vi "RT Connection.vi"(9 "Next State in":T1, 10 "reader endpoint":refnum<k21>, 11 "writer endpoint":refnum<k21>) -> (1 "Next State out":T1)   [LabVIEW 2021]
uses:
  Controls/RT Network States.ctl
  <resource>/objmgr/ni.dex.rc
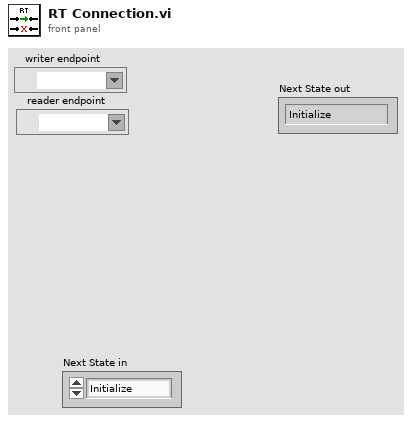
[diagram p1: front panel]
types:
  T1 = typedef "RT Network States.ctl" = enum16{"Initialize", "Connect", "Connected"}
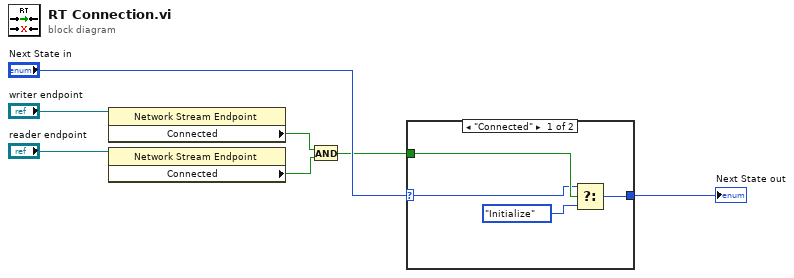
[diagram p0: block diagram]
diagram:
  n1 = property class="Network Stream Endpoint"(reference="writer endpoint") -> ("Connected"=w5:bool)  [unwired: 1 in, 2 out]
  n2 = property class="Network Stream Endpoint"(reference="reader endpoint") -> ("Connected"=w3:bool)  [unwired: 1 in, 2 out]
  n3 = And(x=w5, y=w3) -> (x .and. y?=w1:bool)
  n4 = case shown="\"Connected\"" "Next State in" {
    selector: "Next State in" -> [w8 w12]
    tunnel: [w9 w12] -> w7
    tunnel: w1 -> [w11 _]
    frame "Connected" {
      n5 = Select(t=w8, s=w11, f=RT_Network_States."Initialize" ("Next State in")) -> (s? t:f=w9:T1)
    }
    frame Default {
    }
  }
  "Next State out" <- w7
